vi "ReadData.vi"(5 "ReadNumber":u32, 7 "TimeStamp":timestamp, 8 "error in (no error)":errorcluster, 10 "Data":string) -> (0 "error out":errorcluster, 3 "ReadData":refnum<class "ReadData.lvclass">)   [LabVIEW 2022 SP3, in "Connection.lvlib" / "ReadData.lvclass"]
uses:
  ReadData.lvclass
  ReadData.lvclass/ReadData.ctl
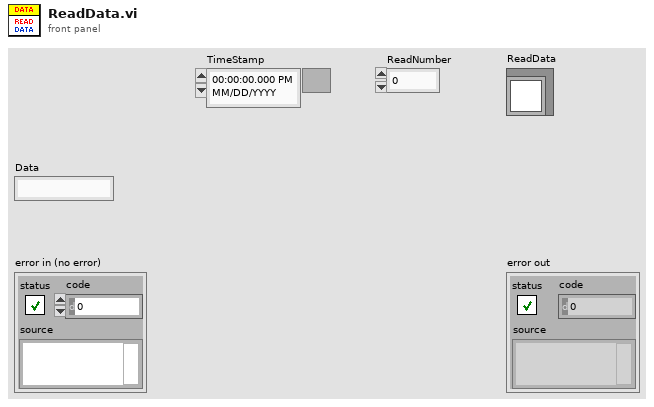
[diagram p1: front panel]
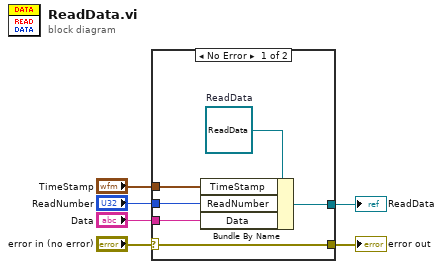
[diagram p0: block diagram]
diagram:
  n1 = case shown="No Error" "error in (no error)" {
    selector: "error in (no error)" -> [w12 w13]
    tunnel: [w12 w13] -> w5
    tunnel: [w7 _] -> w4
    tunnel: "Data" -> [w10 _]
    tunnel: "ReadNumber" -> [w9 _]
    tunnel: "TimeStamp" -> [w8 _]
    frame No Error {
      w11 = refnum<class "ReadData.lvclass"> refnum  # ReadData
      n2 = Bundle By Name(cluster=w11, "TimeStamp"=w8, "ReadNumber"=w9, "Data"=w10) -> (w7:refnum<class "ReadData.lvclass">)
    }
    frame Error {
    }
  }
  "error out" <- w5
  "ReadData" <- w4
